vi "pulse detector on usrp network_controled.vi"() -> ()   [LabVIEW 2021]
doc: "This template is for the Simple NI-USRP Streaming design, a design that shows the basics of streaming data to and from an NI USRP-294x/295x device. Refer to the block diagram for more information about how to use this template."
uses:
  FPGA/reciver params.ctl
  Host/SubVIs/Start Trigger.ctl
  <vilib>/userDefined/Silver/nirio_resource_slv.ctl
  Host/SubVIs/Streaming Xvcr FPGA Ref.ctl
  FPGA/PDW interpoter params.ctl
  Host/SubVIs/Initiate and Fetch (Multi).vi
  Host/SubVIs/Initiate and Fetch Time (Multi).vi
  Host/SubVIs/Initiate and Trigger.vi
  Host/SubVIs/Fetch Rx Data.vi
  Host/SubVIs/Fetch Rx Data (CDB WDT).vi
  Host/SubVIs/Check Aurora Link.vi
  Host/SubVIs/Check Stream Status.vi
  <vilib>/Utility/error.llb/Error Cluster From Error Code.vi
  <vilib>/rvi/errors/niLvFpgaAdjustHostInterfaceError.vi
  <vilib>/rvi/interface/nirviMethod/nirviMethod.xnode
  <vilib>/rvi/interface/nirviReadWriteControl/nirviReadWriteControl.xnode
  <vilib>/FPGAPlugInAG/Dynamic/niLvFpga_ReadFifo_Dynamic.vi
  <vilib>/rvi/errors/niLvFpgaMergeErrorWithErrorCode.vi
  NiFpgaLv.dll
  <vilib>/rvi/interface/Simulation/niFpgaSimulationCallBeginRW.vi
panel:
  in  "save to a file":bool
  in  "Tab Control":enum32{"summary", "Rx graphs"}(tab)
  in  "detection bar (dB)":dbl=85.0 format="%#_3p"
  out "amp(dB)/ frequncy (Hz)":cluster{dbl[], dbl[]}(graph)
  out "amp(dB)":cluster{dbl[], dbl[]}(graph)
  out "F (Hz)":cluster{dbl[], dbl[]}(graph)
  out "PW":cluster{dbl[], dbl[]}(graph)
  out "mun of polses detected":i32
  out "spots from start":i32
  out "pulse rate (PPS)":dbl format="%#_6p"
  in  "base frequnce showen":bool
  in  "sample rate":dbl=200000000.0 format="%#_6p"
  in  "frequency":dbl=800000000.0 format="%#_6p"
  in  "pre amp":dbl=30.0
  in  "PW low bar":dbl
  in  "min AMP":dbl format="%#_3p"
  in  "Pw high bar":dbl=60000.0 format="%#_3g"
  in  "lo likege removal (#of bins)":i32
  out "PW_resolotion":dbl format="%#_6p"
  out "frequncy resolotion":dbl format="%#_3p"
  in  "reciver_params":T1={"min PW (fft cycels)"=0, "max PW (fft cycels)"=1500, "max gap (fft cycels)"=0, "detection bar (liniar amp)"=93.0, "peak detect"=FALSE}
  out "acquiring":bool caption="Streaming"
  in  "Stop":bool
  # "pulse detector on usrp"
  # "this application runs pulse detector on the IQ stream inside the USRP.\nset the parameters and run it.\nthe receiver params are the parameters needed for the pulse detector:\nmax gap - the maximum of undetected parts in the spot that \nthe detector keep looking for continuity.\nRx max PW - if the pulse is CW then we like to get  a PDW even if the pulse isn't done.\nRx min PW - less then this size it's probably just thermal noise\nRx detection bar - the detection bar.\ndisplay filters could help the user make the presenting graphs easier to understand.\npeak detect will reduce the amount of detection related to the pulse skirt, ripples will be delivered as a detections"
  # "AMP"
  # "frequncy"
  # "user filter"
  # "USRP setup"
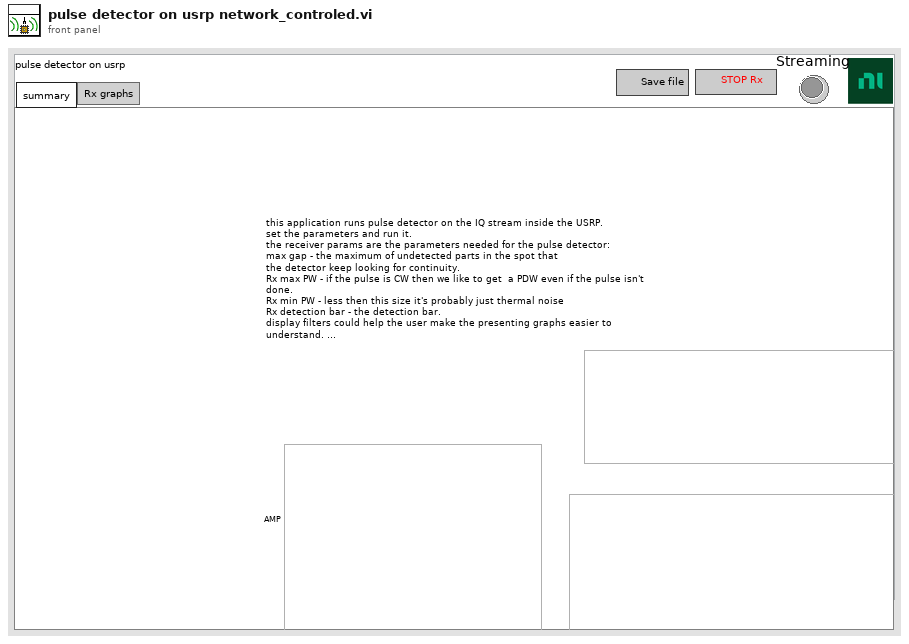
[diagram p1: front panel]
types:
  T1 = typedef "reciver params.ctl" = cluster{"min PW (fft cycels)":u16, "max PW (fft cycels)":u16, "max gap (fft cycels)":u8, "detection bar (liniar amp)":fxp<+,64,63>, "peak detect":bool}
  T2 = typedef "nirio_resource_slv.ctl" = tag
  T3 = typedef "Start Trigger.ctl" = enum8{"Software", "Digital Edge", "Rx Start Trigger", "Tx Start Trigger", "Immediate", "Future Time Event"}
  T4 = cluster{"rf enable 0":bool, "rf config 0":cluster{"antenna":string, "frequency":dbl, "lo frequency":dbl, "level":dbl}, "rf enable 1":bool, "rf config 1":cluster{"antenna":string, "frequency":dbl, "lo frequency":dbl, "level":dbl}, "transfer mode":enum16{"Finite", "Continuous"}, "sample rate":dbl, "number of samples":u32, "start trigger":T3}
  T5 = enum16{"open", "open or create", "create or replace", "create", "open (read-only)"}
  T6 = typedef "Rx Channels.ctl" = cluster{"rx config":cluster{"channel configuration":cluster{"channel enable":bool, "channel configuration":cluster{"antenna":string, "frequency":dbl, "lo frequency":dbl, "level":dbl}}[], "transfer mode":enum16{"Finite", "Continuous"}, "sample rate":dbl, "number of samples":u32, "start trigger":T3}, "reference frequency source":string, "rx.data sink":enum16{"SFP Port 0", "SFP Port 1", "Host"}, "rx.enabled channels":string[], "vertical range":dbl[], "rx.coerced configurations":cluster{"coerced frequencies":dbl[], "coerced lo frequencies":dbl[], "coerced levels":dbl[], "coerced sample rates":dbl[]}}
  T7 = typedef "niUsrpRio Config v1 Host.lvlib/niUsrpRio Session.ctl" = cluster{"FPGA Interface":refnum<k20>, "RIO Interface Number":u32, "Data Clock Rate":u32, "FPGA Data Clock Rate":u32, "Global Settings Register Bus":T8, "Radio 0 Settings Register Bus":T8, "Radio 1 Settings Register Bus":T8, "Radio Settings Bus Semaphore":T9, "DB Queues":T10[], "Characterization Data Valid?":bool, "EEPROM Header":T11, "Device Data Header":T12, "EEPROM Characterization Header":T13, "Characterization Data":T14[], "FPGA Current Version":u32, "FPGA Oldest Compatible Version":u32, "Fixed Logic Current Version":u32, "Fixed Logic Oldest Compatible Version":u32, "FPGA Radio Settings Bus Current Version":u32, "FPGA Radio Settings Bus Oldest Compatible Version":u32, "FPGA Board Config Current Version":u32, "FPGA Board Config Oldest Compatible Version":u32, "Daughterboard Clock Rate":u32, "daughterboard configuration session handles":u64[]}
  T8 = typedef "niInstr Register Bus v0 Host.lvlib/Register Bus Session.ctl" = refnum<queue>
  T9 = typedef "Semaphore RefNum" = refnum<k1>
  T10 = typedef "niUsrpRio Config v1 Host.lvlib/DB Queue Reference.ctl" = refnum<queue>
  T11 = typedef "niUsrpRio Config v1 Host.lvlib/EEPROM Header.ctl" = cluster{"Checksum":u32, "Product Code":u16, "Hardware Current Version":u16, "Hardware Oldest Compatible Version":u16, "EEPROM Map Current Version":u16, "EEPROM Map Oldest Compatible Version":u16, "User Password":string, "Pointer to Factory Header":u32, "Pointer to User Header":u32, "Recommended Interval":u16, "Number of Reserved Bytes":i32, "Number of Daughterboards":u8, "Daughterboard IDs":u16[], "Daughterboard Serial Numbers":string[]}
  T12 = typedef "niUsrpRio Config v1 Host.lvlib/EEPROM Device Data Header.ctl" = cluster{"Checksum":u32, "Number of Channels":u8, "Number of Gain Settings":u16[], "Pointer to Characterization Data":u32[], "Number of Reserved Bytes":i32, "Number of Frequencies":u16[]}
  T13 = typedef "niUsrpRio Config v1 Host.lvlib/EEPROM Characterization Header.ctl" = cluster{"Checksum":u32, "Date":timestamp, "Temperature":sgl, "Misc. Info":string, "Pointer to Device Data Header":u32, "Number of Reserved Bytes":i32}
  T14 = typedef "niUsrpRio Config v1 Host.lvlib/Characterization Data.ctl" = cluster{"Gains[dB]":dbl[], "Frequencies [Hz]":dbl[], "IQ Imbalance Table":T15[], "Measured Gains[dB]":dbl[][]}
  T15 = typedef "niUsrpRio Config v1 Host.lvlib/IQ Imbalance.ctl" = cluster{"Gain Imbalance [linear]":dbl, "Phase Imbalance [radians]":dbl, "Offset":cdb}
  T16 = typedef "PDW interpoter params.ctl" = cluster{"Fs (Hz)":u32, "fft size ":u32, "F base (Hz)":u32, "min AMP (dB)":dbl, "PW low bar (fft cycle)":dbl, "Pw high bar (fft cycle)":dbl, "lo likege removal (fft bin)":i32, "max gap (fft cycle)":dbl}
  T17 = typedef "Streaming Xvcr FPGA Ref.ctl" = refnum<k20>
  T18 = cluster{"rx.state":enum16{"Idle", "Active"}, "rx.samples processed":u32, "rx.number of fifo overflows":u32, "rx.number of iq data overflows":u64[], "rx.dsp reset done":bool}
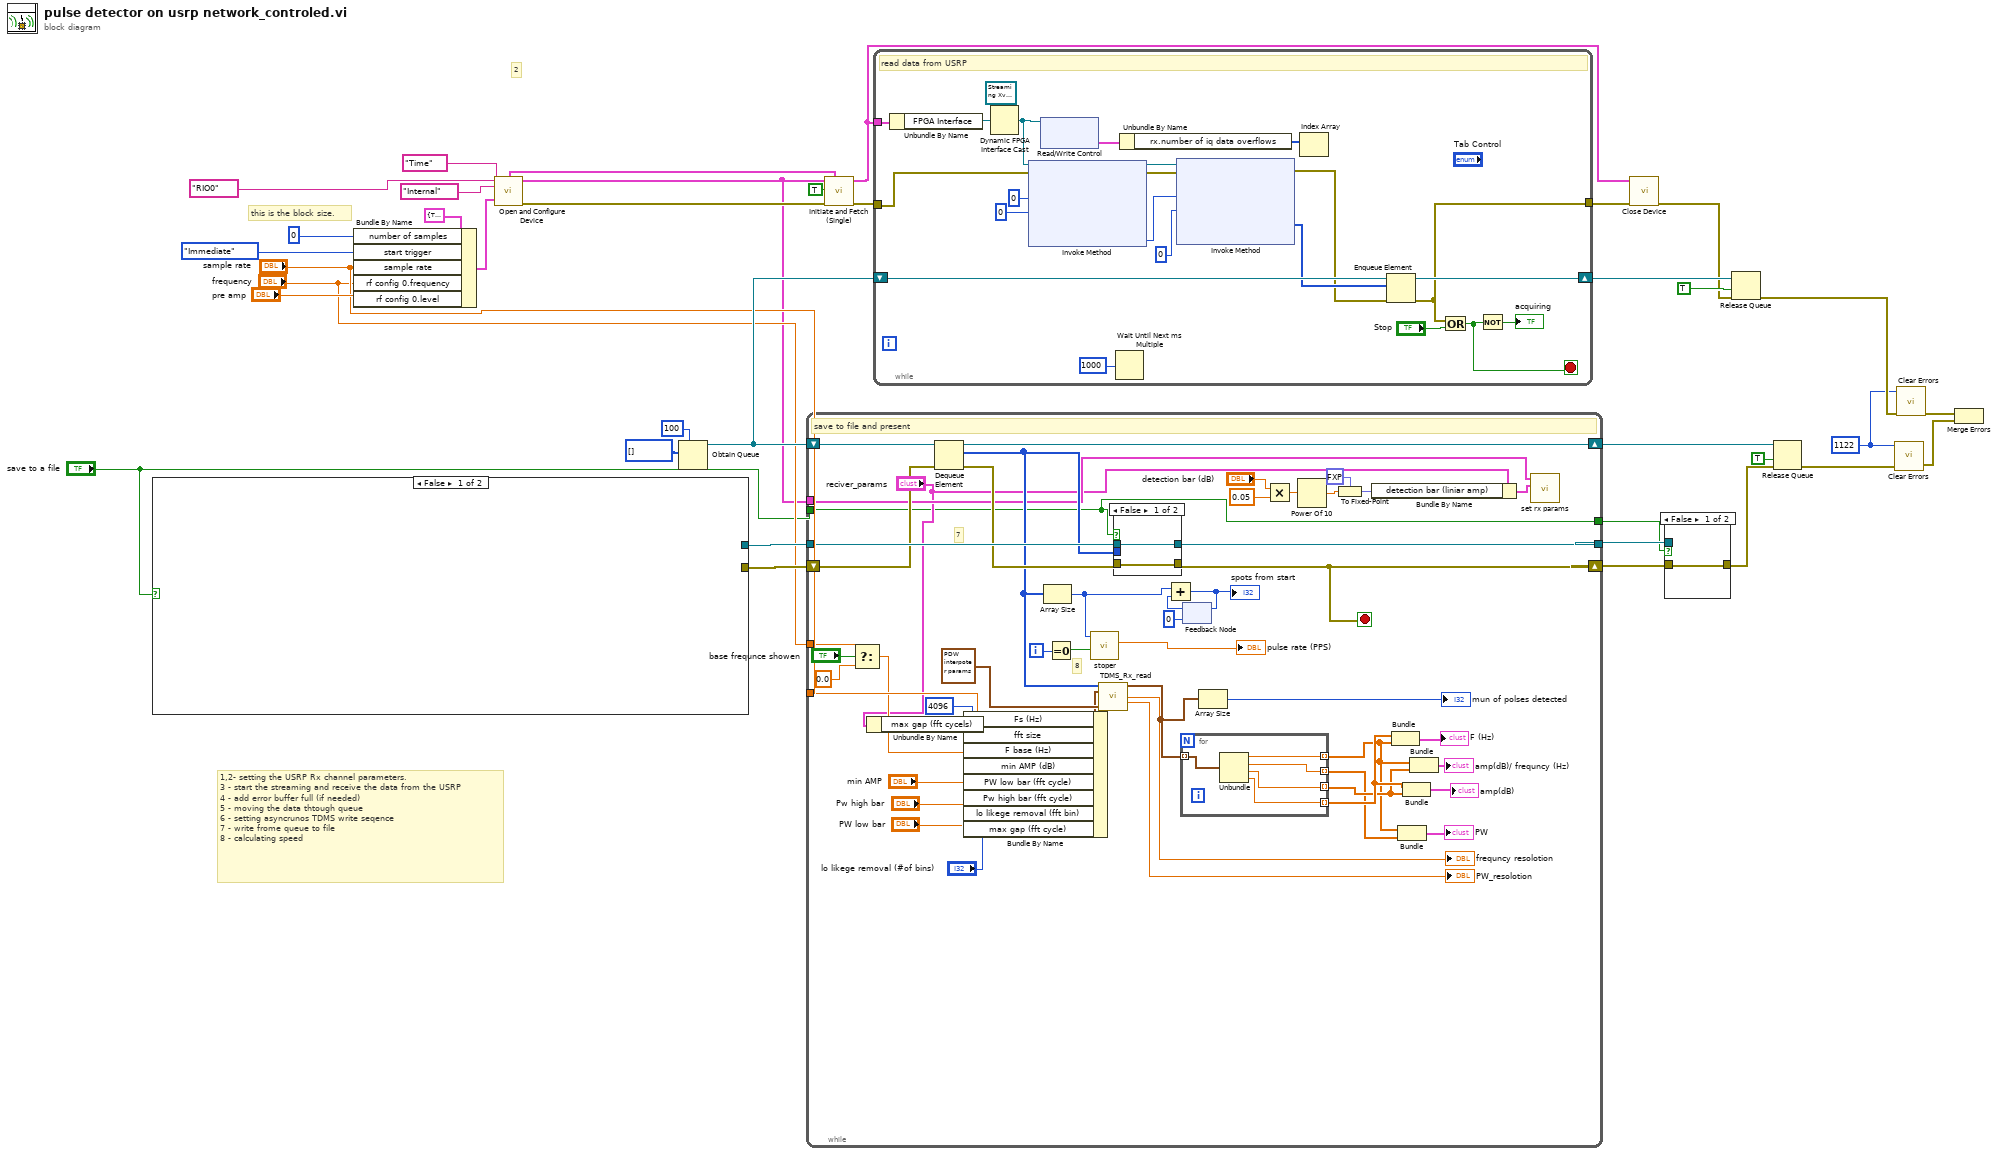
[diagram p0: block diagram]
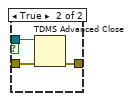
[diagram p2: hidden frame]
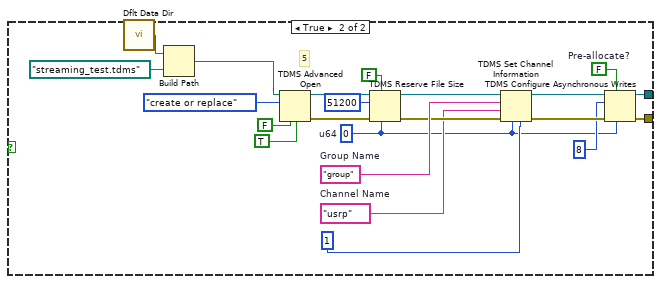
[diagram p3: hidden frame]
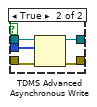
[diagram p4: hidden frame]
diagram:
  w23 = 1122 ("specific error code to clear (0: all)")
  # "2"
  # "this is the block size."
  # "1,2- setting the USRP Rx channel parameters.\n3 - start the streaming and receive the data from the USRP\n4 - add error buffer full (if needed)\n5 - moving the data thtough queue   \n6 - setting asyncrunos TDMS write seqence\n7 - write frome queue to file\n8 - calculating speed"
  n1 = case shown="False" "save to a file" {
    tunnel: [_ w47] -> w37
    tunnel: [_ w46] -> w34
    frame False {
    }
    frame True {
      w50 = FALSE  # Pre-allocate?
      w43 = u64 0  # u64
      w59 = "group"  # Group Name
      w45 = "usrp"  # Channel Name
      # "5"
      n2 = call <vilib>:"Dflt Data Dir.vi"() -> ("App:Default Data Directory"=w40:path)
      n3 = Build Path(base path=w40, name or relative path=path "streaming_test.tdms") -> (appended path=w39:path)
      n4 = TDMS Advanced Open(4:TRUE ("enable asynchronous? (T)"), 6:FALSE ("disable buffering? (T)"), 10:T5."create or replace" ("operation (0:open)"), 11:w39) -> (0:w55:errorcluster, 3:w56:refnum<k34>)  [unwired: 1 in, 1 out]
      n5 = TDMS Reserve File Size(6:w43, 7:FALSE ("append? (T)"), 8:w55, 10:u64 51200 ("reserve size"), 11:w56) -> (0:w53:errorcluster, 3:w54:refnum<k34>)
      n6 = TDMS Set Channel Information(4:u32 1 ("y"), 6:w43, 8:w53, 9:w45, 10:w59, 11:w54) -> (0:w52:errorcluster, 3:w51:refnum<k34>)  [unwired: 1 in]
      n7 = TDMS Configure Asynchronous Writes(6:w43, 7:w50, 8:w52, 10:u32 8 ("max asynchronous writes (4)"), 11:w51) -> (0:w46:errorcluster, 3:w47:refnum<k34>)  [unwired: 2 in]
    }
  }
  n8 = Bundle By Name(cluster=T4 {"rf enable 0"=TRUE, "rf config 0"={"antenna"="RX1", "frequency"=2000000000.0, "lo frequency"=-1.0, "level"=0.0}, "rf enable 1"=FALSE, "rf config 1"={"antenna"="RX2", "frequency"=2000000000.0, "lo frequency"=-1.0, "level"=0.0}, "transfer mode"=enum."Continuous", "sample rate"=10000000.0, "number of samples"=4194304, "start trigger"=enum."Immediate"} ("rx config"), "number of samples"=0, "start trigger"=Start_Trigger."Immediate", "sample rate"="sample rate", "rf config 0.frequency"="frequency", "rf config 0.level"="pre amp") -> (w16:T4)
  n9 = call "Open and Configure Device.vi"("USRP RIO Device"=T2 "RIO0" ("USRP RIO device"), "reference frequency source"="Internal", "which bitfile"="Time", "rx config"=w16) -> ("rx channels"=w10:T6, "niUsrpRio Session (out)"=w3:T7, "error out"=w4:errorcluster)  [unwired: 5 in, 4 out]
  n10 = Obtain Queue(max queue size (-1, unlimited)=100, element data type=u64[] [] ("waveform data")) -> (queue out=w24:refnum<queue>)  [unwired: 3 in, 2 out]
  n11 = while {
    tunnel: w37 -> [w108]
    shift-right: [w104] -> w35
    shift-left: w24 -> [w109]
    tunnel: [w106] -> w36
    shift-right: [w107] -> w33
    shift-left: w34 -> [w103]
    tunnel: "sample rate" -> [w74]
    tunnel: "frequency" -> [w72]
    tunnel: w3 -> [w65]
    tunnel: "save to a file" -> [w60]
    tunnel: [w60] -> w1
    i -> [w105]
    stop <- w107 stop-if-true
    # "8"
    # "7"
    # "save to file and present"
    n12 = Select(t=w72, s="base frequnce showen", f=0.0) -> (s? t:f=w73:dbl)
    n13 = Unbundle By Name("reciver_params") -> ("max gap (fft cycels)"=w79:u8)
    n14 = Dequeue Element(queue=w109, error in (no error)=w103) -> (queue out=w104:refnum<queue>, element=w84:u64[], error out=w102:errorcluster)  [unwired: 1 in, 1 out]
    n15 = Bundle By Name(cluster=T16 {"Fs (Hz)"=200000000, "fft size "=4096, "F base (Hz)"=2000000000, "min AMP (dB)"=0.0, "PW low bar (fft cycle)"=0.0, "Pw high bar (fft cycle)"=7000.0, "lo likege removal (fft bin)"=-1, "max gap (fft cycle)"=0.0} ("PDW interpoter params"), "Fs (Hz)"=w74, "fft size"=u32 4096, "F base (Hz)"=w73, "min AMP (dB)"="min AMP", "PW low bar (fft cycle)"="PW low bar", "Pw high bar (fft cycle)"="Pw high bar", "lo likege removal (fft bin)"="lo likege removal (#of bins)", "max gap (fft cycle)"=w79) -> (w81:T16)
    n16 = Array Size(array=w84) -> (size(s)=w99:i32)
    n17 = Equal To 0?(x=w105) -> (x = 0?=w101:bool)
    n18 = call "stoper.vi"("start"=w101, "x mission"=w99) -> ("x rate"=→"pulse rate (PPS)":dbl)  [unwired: 7 in, 2 out]
    n19 = call "TDMS_Rx_read.vi"("Array in"=w84, "PDW interpoter params"=w81) -> ("Array"=w85:cluster{dbl, dbl, "fixed-point":dbl, dbl}[], "frequncy resolotion"=→"frequncy resolotion":dbl, "PW_resolotion"=→"PW_resolotion":dbl)  [unwired: 11 in]
    n20 = case shown="False" w60 {
      tunnel: w108 -> [w110 w116]
      tunnel: [w111 w115] -> w107
      tunnel: [w110 w114] -> w106
      tunnel: w102 -> [w111 w113]
      tunnel: w84 -> [_ w112]
      frame False {
      }
      frame True {
        n21 = TDMS Advanced Asynchronous Write(8:w113, 10:w112, 11:w116) -> (0:w115:errorcluster, 3:w114:refnum<k34>)
      }
    }
    n22 = for {
      tunnel: w85 -> [w121] mode=indexing
      tunnel: [w120] -> w83 mode=indexing
      tunnel: [w119] -> w86 mode=indexing
      tunnel: [w118] -> w87 mode=indexing
      tunnel: [w117] -> w88 mode=indexing
      n23 = Unbundle(w121) -> (w120:dbl, w119:dbl, "fixed-point"=w118:dbl, w117:dbl)
    }
    n24 = feedback #1(0) -> (w97:i32)
    n25 = Add(x=w99, y=w97) -> (x+y=w98:i32)
    "spots from start" <- w98
    n26 = feedback-in #1(w98) -> ()
    n27 = Array Size(array=w85) -> (size(s)=→"mun of polses detected":i32)
    n28 = Multiply(x="detection bar (dB)", y=0.05) -> (x*y=w66:dbl)
    n29 = Power Of 10(x=w66) -> (10^x=w67:dbl)
    n30 = To Fixed-Point(fixed-point type=fxp<+,64,63> 0.0 ("detection bar (liniar amp)"), number=w67) -> (fixed-point=w68:fxp<+,64,63>)
    n31 = Bundle By Name(cluster="reciver_params", "detection bar (liniar amp)"=w68) -> (w69:T1)
    n32 = Bundle(w88, w83) -> (→"F (Hz)":cluster{dbl[], dbl[]})  [unwired: 1 in]
    n33 = Bundle(w83, w86) -> (→"PW":cluster{dbl[], dbl[]})  [unwired: 1 in]
    n34 = Bundle(w88, w87) -> (→"amp(dB)":cluster{dbl[], dbl[]})  [unwired: 1 in]
    n35 = Bundle(w83, w87) -> (→"amp(dB)/ frequncy (Hz)":cluster{dbl[], dbl[]})  [unwired: 1 in]
    n36 = call "set rx params.vi"("reciver_params"=w69, "niUsrpRio Session (out)"=w65) -> ()  [unwired: 8 in, 2 out]
  }
  n37 = call "Initiate and Fetch (Single).vi"("niUsrpRio Session"=w3, "rx channels"=w10, "first iteration"=TRUE, "error in"=w4) -> ("niUsrpRio Session (out)"=w9:T7, "error out"=w8:errorcluster)  [unwired: 9 in, 1 out]
  n38 = while {
    shift-right: [w143] -> w30
    shift-left: w24 -> [w142]
    tunnel: [w138] -> w14
    tunnel: w9 -> [w133]
    tunnel: w8 -> [w125]
    stop <- w139 stop-if-true
    # "read data from USRP"
    n39 = Unbundle By Name(w133) -> ("FPGA Interface"=w137:refnum<k20>)
    n40 = Dynamic FPGA Interface Cast(Session In=T17 refnum ("Type"), Type=w137) -> (Session Out=w127:T17)
    n41 = xnode "Invoke Method"("FPGA VI Reference In"=w127, "error in"=w125, "Number of Elements"=u32 0, "Timeout (ms)"=0) -> ("FPGA VI Reference Out"=w123:T17, "error out"=w126:errorcluster, "Elements Remaining"=w132:u32)  [unwired: 1 out]
    n42 = xnode "Read/Write Control"("FPGA VI Reference In"=w127) -> ("rx.status"=w135:T18)  [unwired: 1 in, 2 out]
    n43 = Wait Until Next ms Multiple(millisecond multiple=u32 1000) -> ()  [unwired: 1 out]
    n44 = Unbundle By Name(w135) -> ("rx.number of iq data overflows"=w134:u64[])
    n45 = xnode "Invoke Method"("FPGA VI Reference In"=w123, "error in"=w126, "Number of Elements"=w132, "Timeout (ms)"=0) -> ("error out"=w124:errorcluster, "Data"=w129:u64[])  [unwired: 2 out]
    n46 = Index Array(array=w134) -> ()  [unwired: 1 in, 1 out]
    n47 = Enqueue Element(queue=w142, element=w129, error in (no error)=w124) -> (queue out=w143:refnum<queue>, error out=w138:errorcluster)  [unwired: 1 in, 1 out]
    n48 = Or(x=w138, y="Stop") -> (x .or. y?=w139:bool)
    n49 = Not(x=w139) -> (.not. x?=→"acquiring":bool)
  }
  n50 = call "Close Device.vi"("niUsrpRio Session"=w9, "error in"=w14) -> ("error out"=w15:errorcluster)  [unwired: 13 in]
  n51 = case shown="False" w1 {
    tunnel: w36 -> [_ w147]
    tunnel: w33 -> [w144 w146]
    tunnel: [w144 w145] -> w31
    frame False {
    }
    frame True {
      n52 = TDMS Advanced Close(8:w146, 11:w147) -> (0:w145:errorcluster)  [unwired: 2 in, 1 out]
    }
  }
  n53 = Release Queue(queue=w30, force destroy? (F)=TRUE, error in (no error)=w15) -> (error out=w26:errorcluster)  [unwired: 2 out]
  n54 = Release Queue(queue=w35, force destroy? (F)=TRUE, error in (no error)=w31) -> (error out=w25:errorcluster)  [unwired: 2 out]
  n55 = call <vilib>:"Clear Errors.vi"("error in (no error)"=w25, "specific error code to clear (0: all)"=w23) -> ("error out"=w22:errorcluster)  [unwired: 4 in, 1 out]
  n56 = call <vilib>:"Clear Errors.vi"("error in (no error)"=w26, "specific error code to clear (0: all)"=w23) -> ("error out"=w27:errorcluster)  [unwired: 4 in, 1 out]
  n57 = Merge Errors(w27, w22) -> ()  [unwired: 1 out]
